vi "Heat_Tape_Status.vi"() -> (1 "n_ng":u8, 2 "values":T1)   [LabVIEW 2019]
uses:
  Heat_Tape_Global.vi
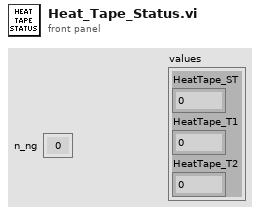
[diagram p1: front panel]
types:
  T1 = cluster{"HeatTape_ST":u32, "HeatTape_T1":dbl, "HeatTape_T2":dbl}
  T2 = enum32{"Bad", "Idle", "Run top level", "Running"}
  T3 = cluster{"MKS670_1000_ST":u32, "HeatTape_T1":dbl, "HeatTape_T2":dbl}
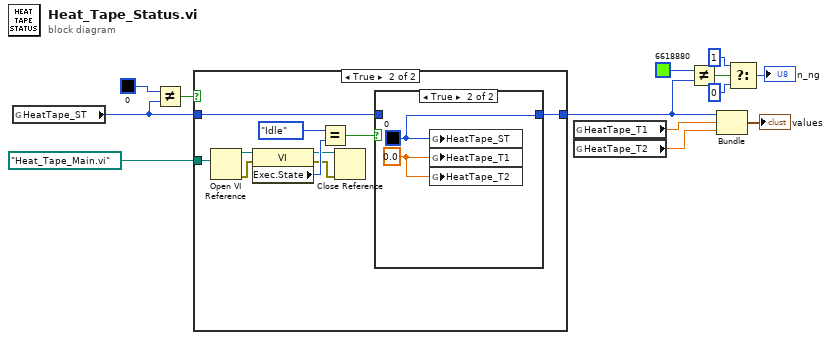
[diagram p0: block diagram]
diagram:
  n1 = global read "Heat_Tape_Global.vi" "HeatTape_ST"() -> (w4:u32)
  n2 = Not Equal?(x=u32 0 ("MKS670_1000_ST 2"), y=w4) -> (x != y?=w13:bool)
  n3 = case shown="True" w13 {
    tunnel: w4 -> [w14 w16]
    tunnel: [w14 w15] -> w10
    tunnel: path "Heat_Tape_Main.vi" ("vi path") -> [_ w17]
    frame False {
    }
    frame True {
      n4 = Open VI Reference(vi path=w17) -> (vi reference=w24:refnum<vi>, error out=w23:errorcluster)  [unwired: 5 in]
      n5 = property class="VI"(reference=w24, error in=w23) -> (reference out=w19:refnum<vi>, error out=w18:errorcluster, "Exec.State"=w21:T2)
      n6 = Equal?(x=T2."Idle" ("Execution:State"), y=w21) -> (x = y?=w22:bool)
      n7 = Close Reference(reference=w19, error in (no error)=w18) -> ()  [unwired: 1 out]
      n8 = case shown="True" w22 {
        tunnel: w16 -> [w25 _]
        tunnel: [w25 w27] -> w15
        frame False {
        }
        frame True {
          w26 = 0.0 ("MKS670_1000_P")
          w27 = u32 0 ("MKS670_1000_ST")
          n9 = global write "Heat_Tape_Global.vi" "HeatTape_ST"(w27) -> ()
          n10 = global write "Heat_Tape_Global.vi" "HeatTape_T1"(w26) -> ()
          n11 = global write "Heat_Tape_Global.vi" "HeatTape_T2"(w26) -> ()
        }
      }
    }
  }
  n12 = global read "Heat_Tape_Global.vi" "HeatTape_T1"() -> (w3:dbl)
  n13 = global read "Heat_Tape_Global.vi" "HeatTape_T2"() -> (w2:dbl)
  n14 = Not Equal?(x=u32 6618880 ("MKS670_1000_ST 2"), y=w10) -> (x != y?=w8:bool)
  n15 = Bundle("MKS670_1000_ST"=w10, "HeatTape_T1"=w3, "HeatTape_T2"=w2) -> (→"values":T3)  [unwired: 1 in]
  n16 = Select(t=u8 1 ("n_ng"), s=w8, f=u8 0 ("n_ng")) -> (s? t:f=→"n_ng":u8)
